vi "Write ROI Descriptor.vi"(8 "error in (no error)":errorcluster, 10 "ROI Descriptor":T1 {"Contours"."Type" items=["No Selection", "Point", "Line", "Rectangle", "Oval", "Polygon", "Freehand Region", "Annulus", "Unused2", "Unused3", "Broken Line", "Freehand Line", "Rotated Rectangle"]}, 11 "ROIed Video Frame in":refnum<class "ROIed Video Frame.lvclass">) -> (0 "error out":errorcluster, 3 "ROIed Video Frame out":refnum<class "ROIed Video Frame.lvclass">)   [LabVIEW 2018, in "ROIed Video Frame.lvclass"]
uses:
  ROIed Video Frame.lvclass
  ROIed Video Frame.lvclass/ROIed Video Frame.ctl
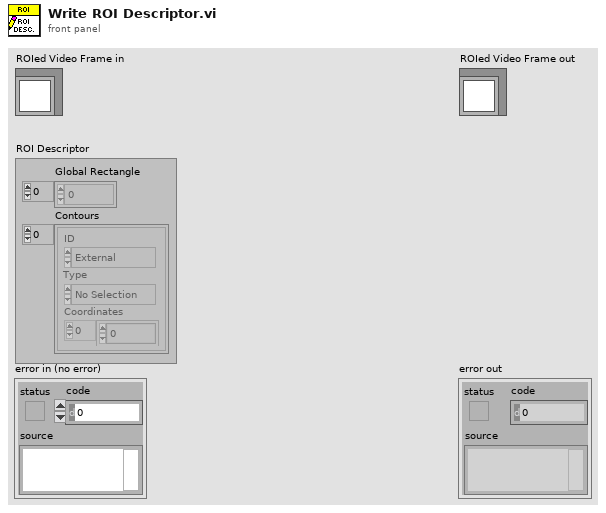
[diagram p1: front panel]
types:
  T1 = typedef "ROI Descriptor" = cluster{"Global Rectangle":i32[], "Contours":cluster{"ID":enum32{"External", "Internal"}, "Type":u32, "Coordinates":i32[]}[]}
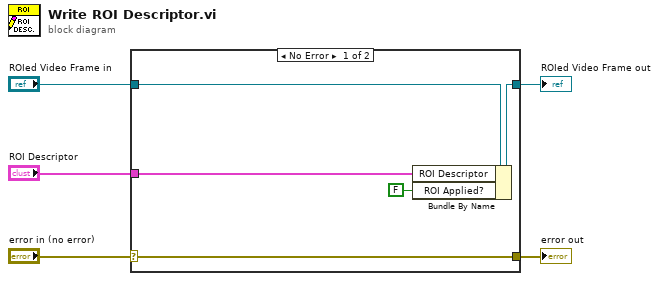
[diagram p0: block diagram]
diagram:
  n1 = case shown="No Error" "error in (no error)" {
    selector: "error in (no error)" -> [w10 w11]
    tunnel: [w10 w11] -> w4
    tunnel: [w8 w12] -> w2
    tunnel: "ROIed Video Frame in" -> [w9 w12]
    tunnel: "ROI Descriptor" -> [w7 _]
    frame No Error {
      n2 = Bundle By Name(cluster=w9, "ROI Descriptor"=w7, "ROI Applied?"=FALSE) -> (w8:refnum<class "ROIed Video Frame.lvclass">)
    }
    frame Error {
    }
  }
  "error out" <- w4
  "ROIed Video Frame out" <- w2
